vi "Waveform Simulator.vi"(9 "Waveform Parameters":T1, 10 "Digitizing Parameters":T2) -> (2 "Waveform Output":cluster{"Time":dbl[], "Displacement":dbl[]})   [LabVIEW 2014]
uses:
  <vilib>/imath/engines/lvmath2/RunTimeEngine/Managers/WorkSpace/UID Generator.vi
  <vilib>/imath/engines/lvmath2/RunTimeEngine/RunTimeType/NIMS_RunTimeType_From StrictType (excl LVString).vi
  <instcachedir>/0/NIMS_RunTimeType_From StrictType (excl LVString)_15A5391EEA9C4AACB9955AC755B83D29.lvgen/NIMS_RunTimeType_From StrictType (excl LVString)_15A5391EEA9C4AACB9955AC755B83D29_000.vi
  <vilib>/imath/engines/lvmath2/RunTimeEngine/LocalVariableDefStatement/MC_LocalVariableDefStatement_Display.vi
  <vilib>/imath/engines/lvmath2/RunTimeEngine/RangeToken/NIMS_Range.vi
  <instcachedir>/0/NIMS_Range_9BCE657718DF4976A877346C61F22738.lvgen/NIMS_Range_9BCE657718DF4976A877346C61F22738_000.vi
  <vilib>/imathl/engines/lvmath/Functions/Error Handling/Create Error.vi
  <vilib>/imath/engines/lvmath2/RunTimeEngine/Managers/SymbolTable/Clear UID.vi
  <vilib>/imath/engines/lvmath2/RunTimeEngine/NodeEndStatement/NIMS_NodeEndStatement_Output.vi
  <instcachedir>/0/NIMS_NodeEndStatement_Output_53EC0D466D134D7ABD903AC30B43404B.lvgen/NIMS_NodeEndStatement_Output_53EC0D466D134D7ABD903AC30B43404B_005.vi
  <vilib>/imath/engines/lvmath2/RunTimeEngine/ErrorHandling/NIMS_Finalize Error.vi
  <vilib>/imath/engines/lvmath2/RunTimeEngine/Managers/SymbolTable/NIMS_WorkSpace.lvlib
panel:
  out "XY Graph":cluster{"t":dbl[], "x":dbl[]}(graph)
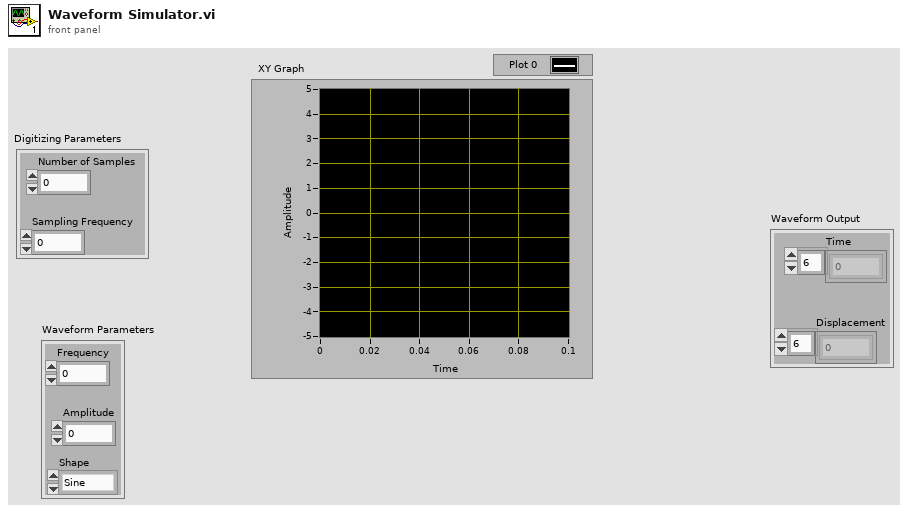
[diagram p1: front panel]
types:
  T1 = cluster{"Frequency":dbl, "Amplitude":dbl, "Shape":enum16{"Sine", "Cosine", "DC Level", "Square", "User-Defined"}}
  T2 = cluster{"Number of Samples":i32, "Sampling Frequency":dbl}
  T3 = enum16{"Sine", "Cosine", "DC Level", "Square", "User-Defined"}
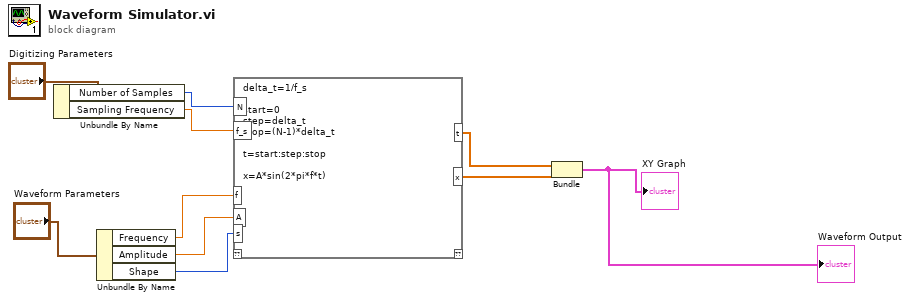
[diagram p0: block diagram]
diagram:
  n1 = Unbundle By Name("Digitizing Parameters") -> ("Number of Samples"=w5:i32, "Sampling Frequency"=w4:dbl)
  n2 = Unbundle By Name("Waveform Parameters") -> ("Frequency"=w9:dbl, "Amplitude"=w8:dbl, "Shape"=w7:T3)
  n3 = mathscript code="delta_t=1/f_s\n\nstart=0\nstep=delta_t\nstop=(N-1)*delta_t\n\nt=start:step:stop\n\nx=A*sin(2*pi*f*t)"("f"=w9, "A"=w8, "s"=w7, "N"=w5, "f_s"=w4) -> ("t"=w3:dbl[], "x"=w2:dbl[])  [unwired: 1 in, 1 out]
  n4 = Bundle("t"=w3, "x"=w2) -> (→"XY Graph" →"Waveform Output":cluster{"t":dbl[], "x":dbl[]})  [unwired: 1 in]
